vi "button actuation counter.vi"(0 "old count":i32, 1 "was button pressed ?":bool, 3 "button pressed now":bool) -> (7 "new count":i32)   [LabVIEW 2016]
panel:
  # "RETORNA O NÚMERO DE VEZES QUE A ENTRADA\nMUDA DE FALSE PARA TRUE."
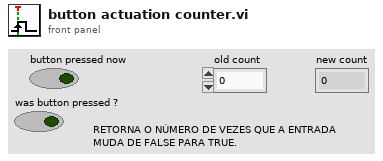
[diagram p1: front panel]
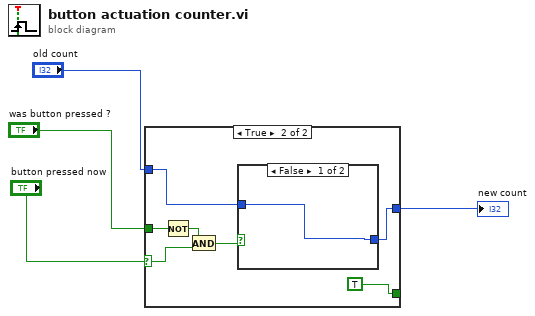
[diagram p0: block diagram]
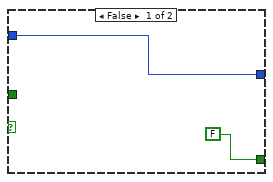
[diagram p2: hidden frame]
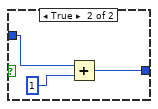
[diagram p3: hidden frame]
diagram:
  n1 = case shown="True" "button pressed now" {
    selector: "button pressed now" -> [_ w8]
    tunnel: "old count" -> [w6 w11]
    tunnel: [w6 w10] -> w4
    tunnel: "was button pressed ?" -> [_ w9]
    tunnel: [FALSE TRUE] -> _
    frame False {
    }
    frame True {
      n2 = Not(x=w9) -> (.not. x?=w12:bool)
      n3 = And(x=w12, y=w8) -> (x .and. y?=w13:bool)
      n4 = case shown="False" w13 {
        tunnel: w11 -> [w14 w16]
        tunnel: [w14 w15] -> w10
        frame False {
        }
        frame True {
          n5 = Add(x=w16, y=1) -> (x+y=w15:i32)
        }
      }
    }
  }
  "new count" <- w4
